vi "VisionFigure.vi"() -> ()   [LabVIEW 2018]
uses:
  <vilib>/vision/Pattern Matching.llb/IMAQ GM Match Report.ctl
panel:
  out "Number of Matches (Pattern Matching 1)":i32
  out "Matches (Pattern Matching 1)":T1[](array[typedef]) {"Correlation Score" format="%.2f"; "Target Template Curve Score" format="%.2f"; "Template Target Curve Score" format="%.2f"; "Bounding Box"."y" format="%.2f"; "Bounding Box"."x" format="%.2f"; "Position"."y" format="%.2f"; "Position"."x" format="%.2f"; "Score" format="%.2f"; "Scale" format="%.2f"; "Angle" format="%.2f"; "Occlusion %" format="%.2f"}
  in  "Stop (F)":bool
  out "Image Out":T2(plugin-control)
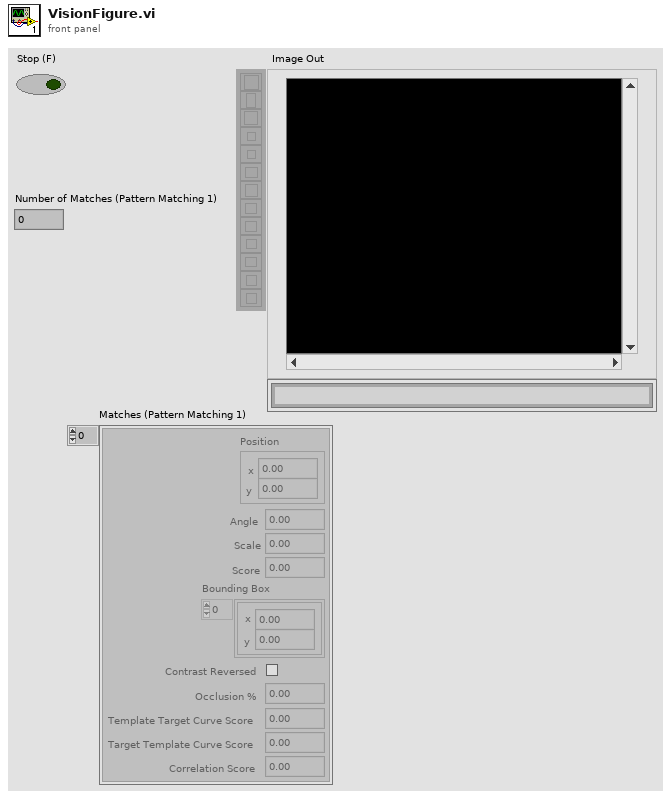
[diagram p1: front panel]
types:
  T1 = typedef "IMAQ GM Match Report.ctl" = cluster{"Position":cluster{"x":sgl, "y":sgl}, "Angle":sgl, "Scale":sgl, "Score":sgl, "Bounding Box":cluster{"x":sgl, "y":sgl}[], "Contrast Reversed":bool, "Occlusion %":sgl, "Template Target Curve Score":sgl, "Target Template Curve Score":sgl, "Correlation Score":sgl}
  T2 = typedef "IMAQ Image.ctl" = refnum<image>
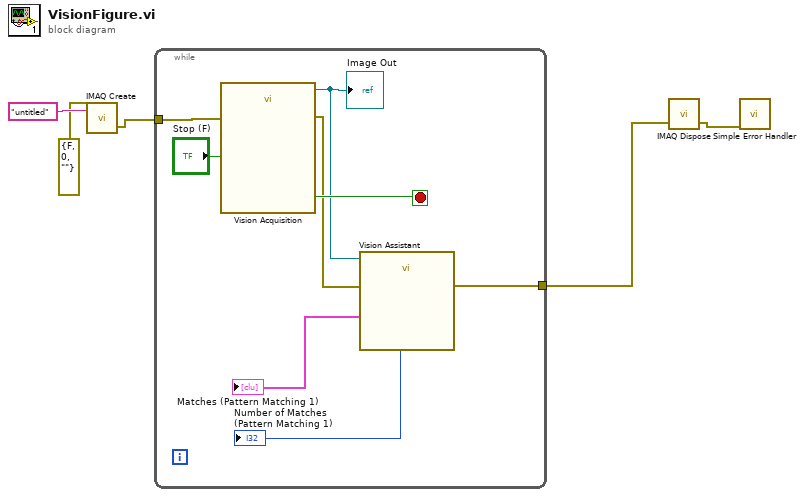
[diagram p0: block diagram]
diagram:
  n1 = call "IMAQ Create"("Image Name"="untitled", "error in (no error)"=errorcluster {"status"=FALSE, "code"=0, "source"=""}) -> ("error out"=w4:errorcluster)  [unwired: 3 in, 1 out]
  n2 = while {
    tunnel: w4 -> [w11]
    tunnel: [w8] -> w1
    stop <- w12 stop-if-true
    n3 = call "Vision Acquisition"("Stop (F)"="Stop (F)", "error in"=w11) -> ("Image Out"=w9:T2, "Stopped"=w12:bool, "error out"=w10:errorcluster)  [unwired: 22 in, 1 out]
    "Image Out" <- w9
    n4 = call "Vision Assistant"("Image In"=w9, "error in"=w10) -> ("Matches (Pattern Matching 1)"=→"Matches (Pattern Matching 1)":T1[], "Number of Matches (Pattern Matching 1)"=→"Number of Matches (Pattern Matching 1)":i32, "error out"=w8:errorcluster)  [unwired: 22 in, 1 out]
  }
  n5 = call "IMAQ Dispose"("error in (no error)"=w1) -> ("error out"=w5:errorcluster)  [unwired: 5 in]
  n6 = call <vilib>:"Simple Error Handler.vi"("error in (no error)"=w5) -> ()  [unwired: 4 in, 5 out]
